vi "I2C_Close.vi"(5 "Bus":i32=1, 8 "error in":errorcluster) -> (0 "error out":errorcluster)   [LabVIEW 2014]
doc: "Read a single byte from the specified I2C device"
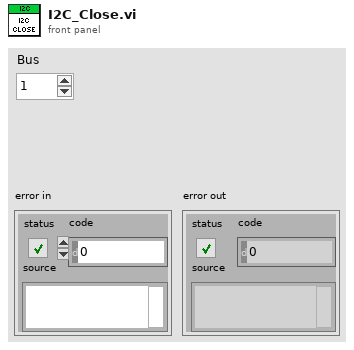
[diagram p1: front panel]
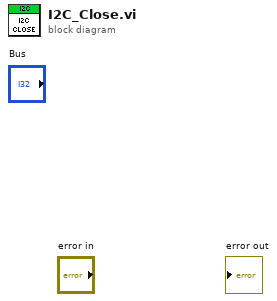
[diagram p0: block diagram]
diagram:
